vi "Process data.vi"(8 "error in (no error)":errorcluster, 11 "Data":variant) -> (0 "error out":errorcluster)   [LabVIEW 2018]
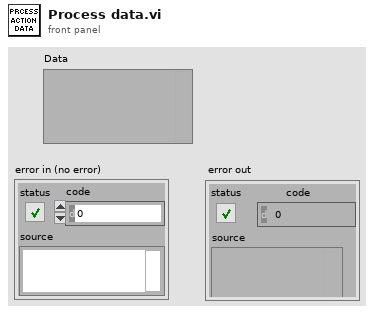
[diagram p1: front panel]
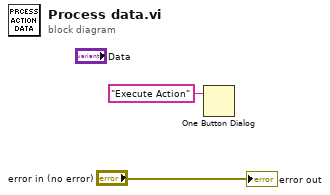
[diagram p0: block diagram]
diagram:
  n1 = One Button Dialog(message="Execute Action") -> ()  [unwired: 1 in, 1 out]
  "error out" <- "error in (no error)"
